vi "GetTrigger (SubVI).vi"(4 "Array in":dbl[][](array[numeric])) -> (1 "Array out":dbl[][](array[numeric]))   [LabVIEW 2017]
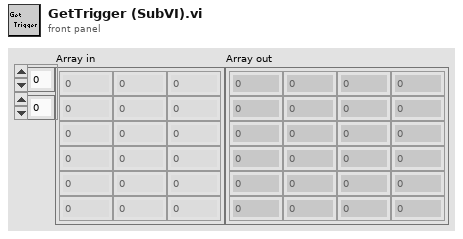
[diagram p1: front panel]
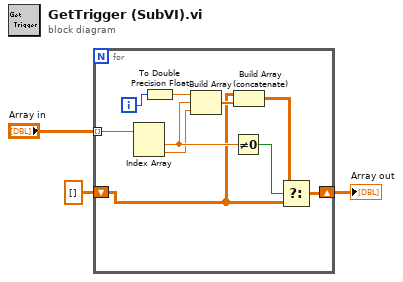
[diagram p0: block diagram]
diagram:
  n1 = for {
    tunnel: "Array in" -> [w13] mode=indexing
    shift-right: [w12] -> w2
    shift-left: dbl[][] [] -> [w4]
    i -> [w10]
    n2 = Index Array(array=w13) -> (element #1=w9:dbl, element #2=w8:dbl)  [unwired: 2 in]
    n3 = To Double Precision Float(number=w10) -> (double precision float=w7:dbl)
    n4 = Build Array(w7, w9, w8) -> (w6:dbl[])
    n5 = Not Equal To 0?(x=w9) -> (x != 0?=w11:bool)
    n6 = Build Array (concatenate)(w4, w6) -> (w5:dbl[][])
    n7 = Select(t=w5, s=w11, f=w4) -> (s? t:f=w12:dbl[][])
  }
  "Array out" <- w2
